vi "C867_Sample_Application_1_RRF.vi"() -> ()   [LabVIEW 2013]
doc: "This VI demonstrates how to define a C-867 configuration with connected axes. In this example the C-867 is connected through COM port 1 with baudrate 38400. The VI runs C867_Multiaxis_Configuration_Setup.vi with these specified settings and reads the position of all axes. The diagram shows how to combine the driver VIs for these tasks.\n\nWarning: Before running this VI, modify Interface and RS232 settings (or add USB settings if Interface = USB was selected) to reflect your configuration. The predefined settings provided with the VI probably do not match your system."
panel:
  in  "stop":bool
  in  "error in":errorcluster
  out "Running":bool caption="C867_Multiaxis_Configuration_Setup.vi is running"
  out "error out":errorcluster
  out "Position":dbl[](array[numeric]) format="%.6f"
  out "Conn. Axes":string[](array[string])
  out "Identification":string
  # "This VI demonstrates how to define a C-867 configuration with a connected axis. In this example the C-867 is connected through \nCOM port 1 with baudrate 38400. The VI runs C867_Multiaxis_Configuration_Setup.vi with these specified settings and reads the \nposition of all axes. The diagram shows how to combine the driver VIs for these tasks. \n\nWarning: Before running this VI, modify \"Interface\", \"RS232 settings\" (or add USB settings if Interface = USB was selected) to reflect\n                 your configuration. The predefined settings provided with the VI probably do not match your system."
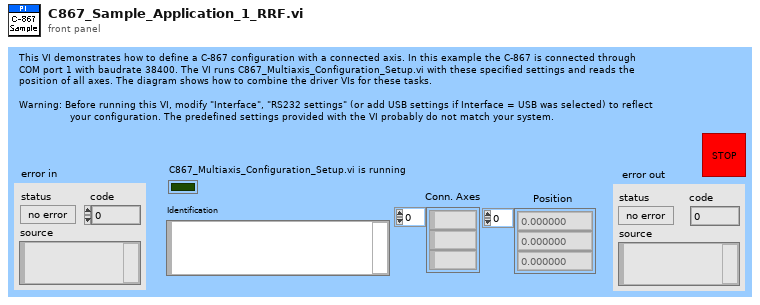
[diagram p1: front panel]
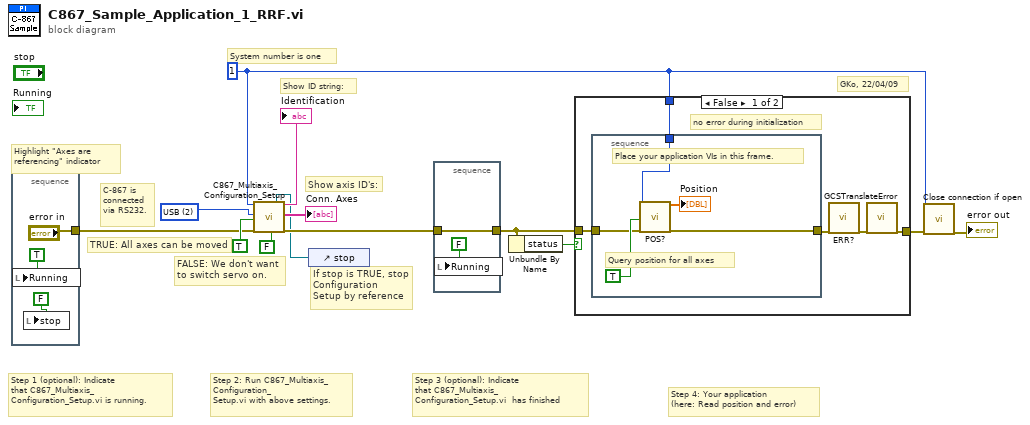
[diagram p0: block diagram]
diagram:
  w1 = u16 2 items=["RS232", "RS232 DaisyChain", "USB"] ("Interface")
  w2 = 1 ("System no.")
  # "C-867 is\nconnected\nvia RS232."
  # "If stop is TRUE, stop \nConfiguration\nSetup by reference"
  # "GKo, 22/04/09"
  # "Step 4: Your application\n(here: Read position and error)"
  # "Step 3 (optional): Indicate\nthat C867_Multiaxis_\nConfiguration_Setup.vi  has finished"
  # "Step 2: Run C867_Multiaxis_\nConfiguration_\nSetup.vi with above settings."
  # "Step 1 (optional): Indicate\nthat C867_Multiaxis_\nConfiguration_Setup.vi is running."
  # "Highlight \"Axes are\nreferencing\" indicator"
  # "Show axis ID's:"
  # "Show ID string:"
  # "FALSE: We don't want\nto switch servo on."
  # "TRUE: All axes can be moved"
  # "System number is one"
  n1 = stacked-sequence {
    tunnel: ["error in"] -> w9
    frame #0 {
      n2 = local write "Running"(TRUE ("Running")) -> ()
      n3 = local write "stop"(FALSE ("stop")) -> ()
    }
  }
  n4 = control-ref of="stop"() -> (w5:refnum<vi>)
  n5 = call "C867_Multiaxis_Configuration_Setup.vi"("System no."=w2, "Interface"=w1, "All axes?"=TRUE, "error in"=w9, "Switch servo on?"=FALSE ("Use dialog to define\nconnected stages?"), "Stop refnum"=w5) -> ("Identification"=→"Identification":string, "Conn. \nAxes"=→"Conn. Axes":string[], "error out"=w10:errorcluster)  [unwired: 7 in, 4 out]
  n6 = stacked-sequence {
    tunnel: w10 -> [w18]
    tunnel: [w18] -> w7
    frame #0 {
      n7 = local write "Running"(FALSE ("Running")) -> ()
    }
  }
  n8 = Unbundle By Name(w7) -> ("status"=w6:bool)
  n9 = case shown="False" w6 {
    tunnel: w2 -> [w23 _]
    tunnel: w7 -> [w22 w29]
    tunnel: [w19 w29] -> w4
    frame False {
      # "no error during initialization"
      n10 = stacked-sequence {
        tunnel: w23 -> [w28]
        tunnel: [w25] -> w20
        tunnel: w22 -> [w24]
        frame #0 {
          # "Place your application VIs in this frame."
          # "Query position for all axes"
          n11 = call "POS?.vi"("System no."=w28, "All axes?"=TRUE, "error in"=w24) -> ("Position"=→"Position":dbl[], "error out"=w25:errorcluster)  [unwired: 15 in]
        }
      }
      n12 = call "ERR?.vi"("error in"=w20) -> ("error out"=w21:errorcluster)  [unwired: 17 in, 1 out]
      n13 = call "GCSTranslateError.vi"("error in"=w21) -> ("error out"=w19:errorcluster)  [unwired: 16 in, 2 out]
    }
    frame True {
      # "error during initialization!"
    }
  }
  n14 = call "Close connection if open.vi"("System no."=w2, "error in"=w4) -> ("error out"=→"error out":errorcluster)  [unwired: 16 in, 1 out]
